vi "EMV Check Limits.vi"(6 "Current Position":dbl, 8 "error in (no error)":errorcluster, 9 "Current Position Slope":dbl, 10 "Previous Position":dbl, 11 "Previous Position Slope":dbl) -> (0 "error out":errorcluster, 2 "Position":dbl, 3 "Slope Output":dbl)   [LabVIEW 2020]
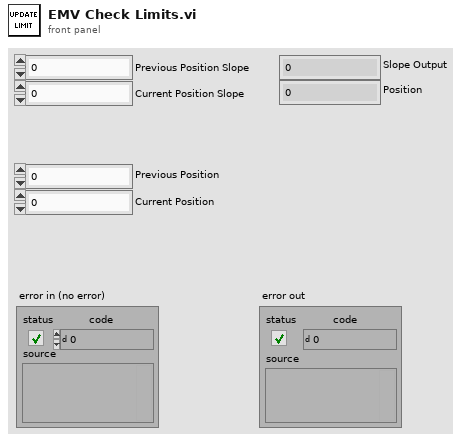
[diagram p1: front panel]
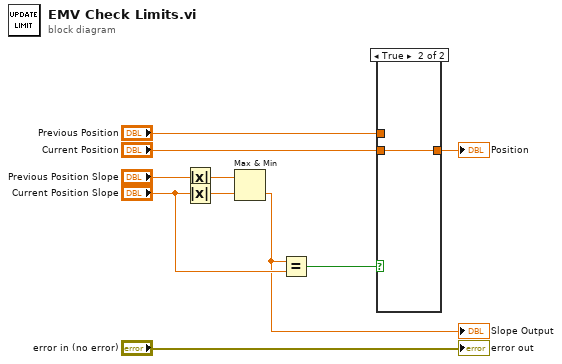
[diagram p0: block diagram]
diagram:
  n1 = Absolute Value(x="Previous Position Slope") -> (abs(x)=w1:dbl)
  n2 = Absolute Value(x="Current Position Slope") -> (abs(x)=w4:dbl)
  n3 = Max & Min(x=w1, y=w4) -> (min(x,y)=w7:dbl)  [unwired: 1 out]
  "Slope Output" <- w7
  n4 = Equal?(x=w7, y="Current Position Slope") -> (x = y?=w5:bool)
  n5 = case shown="True" w5 {
    tunnel: "Current Position" -> [_ w12]
    tunnel: [w11 w12] -> w8
    tunnel: "Previous Position" -> [w11 _]
    frame False {
    }
    frame True {
    }
  }
  "Position" <- w8
  "error out" <- "error in (no error)"
